vi "GetItemsVisible.vi"(8 "error in (no error)":errorcluster, 11 "Tree_LVOOP in":refnum<class "Tree Class.lvclass">) -> (0 "error out":errorcluster, 2 "Visibility Cluster":T1={"Hierarchy Lines"=enum."Visible", "Symbols"=TRUE, "Column Headers"=FALSE, "Row Headers"=FALSE, "Horizontal Lines"=FALSE, "Vertical Lines"=FALSE}, 3 "Tree_LVOOP out":refnum<class "Tree Class.lvclass">)   [LabVIEW 2012, in "Tree Tools.lvlib" / "Tree Class.lvclass"]
uses:
  Tree Class.lvclass
  Tree Class.lvclass/Tree Class.ctl
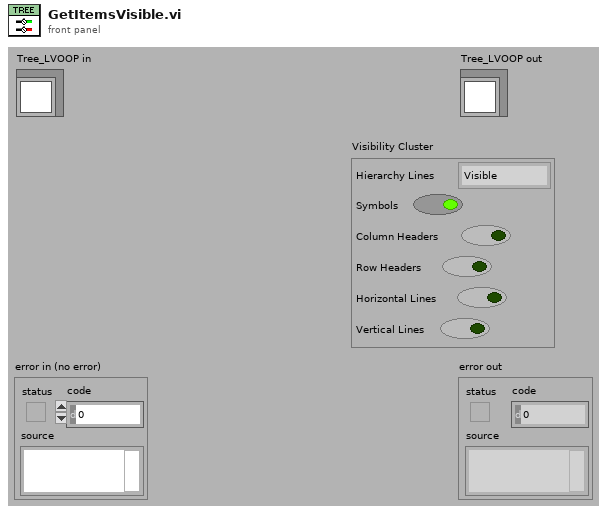
[diagram p1: front panel]
types:
  T1 = cluster{"Hierarchy Lines":enum32{"Visible", "Invisible", "OS Default"}, "Symbols":bool, "Column Headers":bool, "Row Headers":bool, "Horizontal Lines":bool, "Vertical Lines":bool}
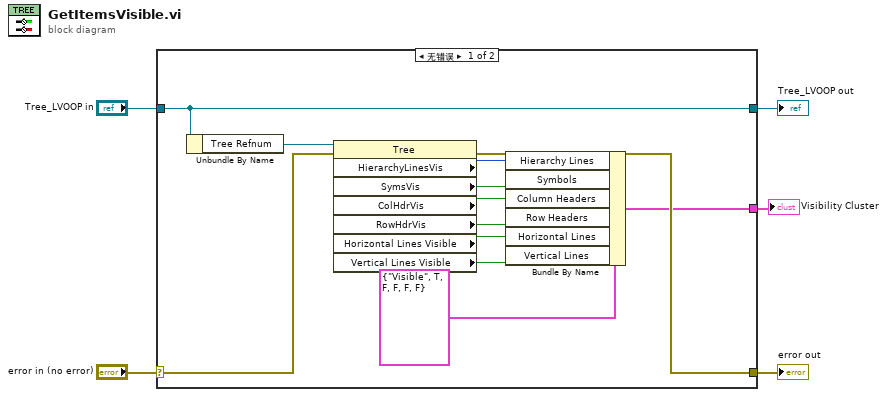
[diagram p0: block diagram]
diagram:
  n1 = case shown="无错误" "error in (no error)" {
    selector: "error in (no error)" -> [w15 w19]
    tunnel: [w14 w19] -> w4
    tunnel: [w17 w18] -> w2
    tunnel: "Tree_LVOOP in" -> [w17 w18]
    tunnel: [w6 _] -> w1
    frame No Error {
      n2 = Unbundle By Name(w17) -> ("Tree Refnum"=w16:refnum<vi>)
      n3 = property class="Tree"(reference=w16, error in=w15) -> (error out=w14:errorcluster, "HierarchyLinesVis"=w12:enum32{"Visible", "Invisible", "OS Default"}, "SymsVis"=w11:bool, "ColHdrVis"=w10:bool, "RowHdrVis"=w9:bool, "Horizontal Lines Visible"=w8:bool, "Vertical Lines Visible"=w7:bool)  [unwired: 1 out]
      n4 = Bundle By Name(cluster=T1 {"Hierarchy Lines"=enum."Visible", "Symbols"=TRUE, "Column Headers"=FALSE, "Row Headers"=FALSE, "Horizontal Lines"=FALSE, "Vertical Lines"=FALSE} ("Visibility Cluster"), "Hierarchy Lines"=w12, "Symbols"=w11, "Column Headers"=w10, "Row Headers"=w9, "Horizontal Lines"=w8, "Vertical Lines"=w7) -> (w6:T1)
    }
    frame Error {
    }
  }
  "error out" <- w4
  "Tree_LVOOP out" <- w2
  "Visibility Cluster" <- w1
